vi "Device Address.vi"(10 "Device":T2=enum."V7") -> (2 "Address (all reqd.)":T1, 3 "Channel Name":string)   [LabVIEW 2011]
uses:
  Valve_Pump.ctl
  ADAM Client/Sub VIs/ADAM Controls/Address.ctl
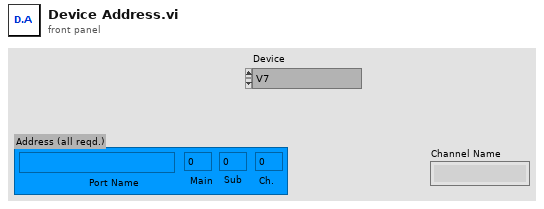
[diagram p1: front panel]
types:
  T1 = typedef "Address.ctl" = cluster{"Main":i32, "Ch.":i32, "Sub":i32, "Port Name":string}
  T2 = typedef "Valve_Pump.ctl" = enum16{"Main Rack Power", "Pump Power", "Valve Power", "V4", "V5", "V6", "V7", "V8", "V9", "V10", "V11", "V12", "V13", "V14", "V15", "V18", "V19", "V20", "V21", "V22", "V23", "V24", "V25", "V26", "V27", "V28", "V29", "V30", "V31", "V32", "V33", "V34", "Pump A", "Pump B", "Pump C", "Pump D"}
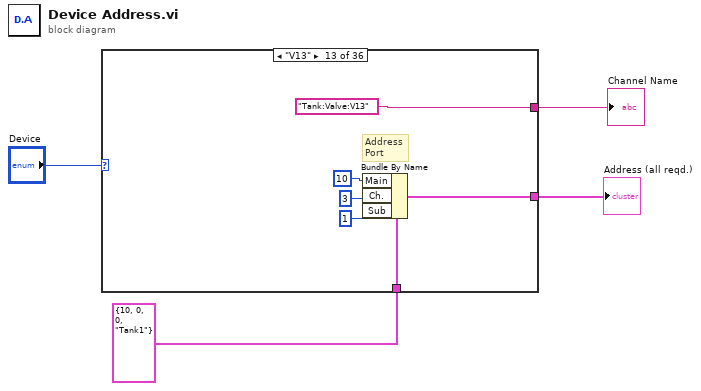
[diagram p0: block diagram]
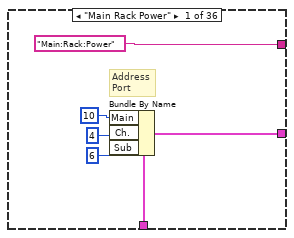
[diagram p2: hidden frame]
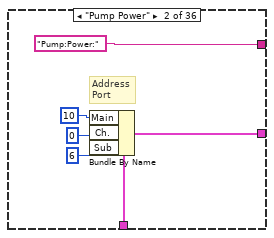
[diagram p3: hidden frame]
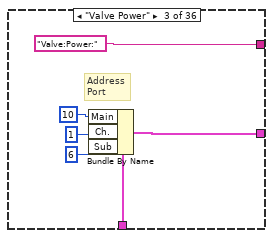
[diagram p4: hidden frame]
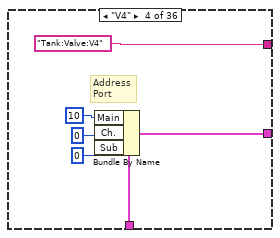
[diagram p5: hidden frame]
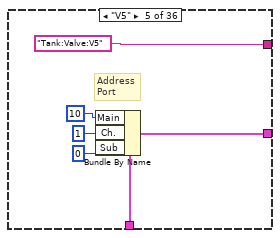
[diagram p6: hidden frame]
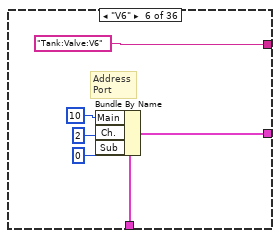
[diagram p7: hidden frame]
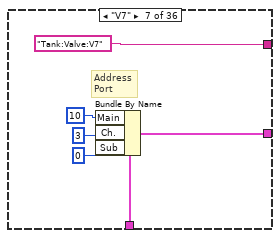
[diagram p8: hidden frame]
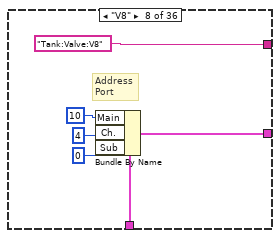
[diagram p9: hidden frame]
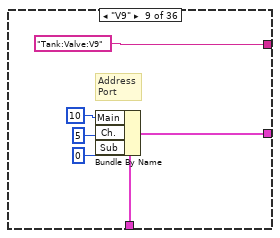
[diagram p10: hidden frame]
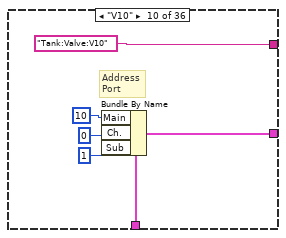
[diagram p11: hidden frame]
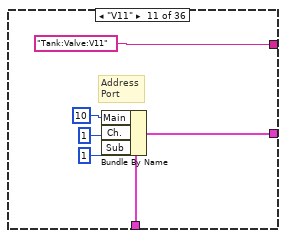
[diagram p12: hidden frame]
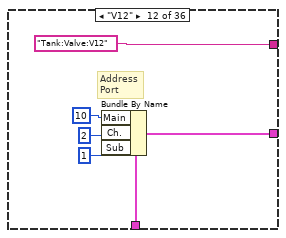
[diagram p13: hidden frame]
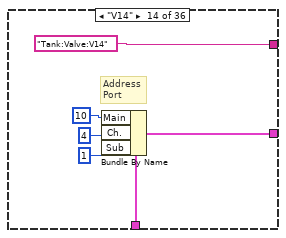
[diagram p14: hidden frame]
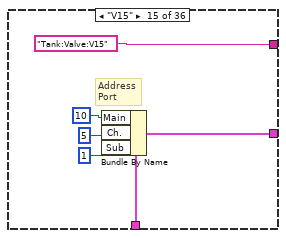
[diagram p15: hidden frame]
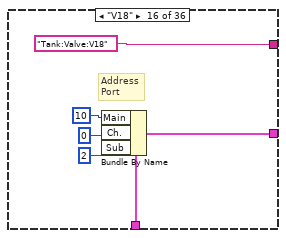
[diagram p16: hidden frame]
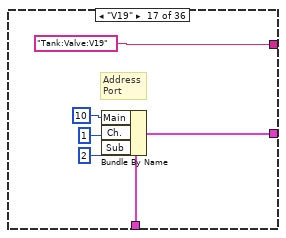
[diagram p17: hidden frame]
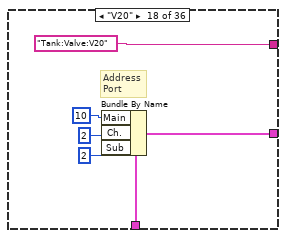
[diagram p18: hidden frame]
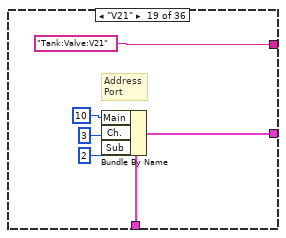
[diagram p19: hidden frame]
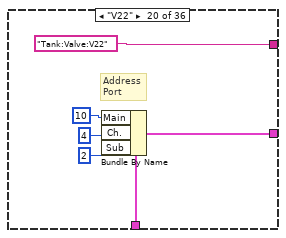
[diagram p20: hidden frame]
diagram:
  n1 = case shown="\"V13\"" "Device" {
    tunnel: T1 {"Main"=10, "Ch."=0, "Sub"=0, "Port Name"="Tank1"} ("Address (all reqd.)") -> [w10 w16 w22 w28 w34 w40 w46 w52 w58 w64 w70 w76 w82 w88 w94 w100 w106 w112 w118 w124 w130 w136 w142 w148 w154 w160 w166 w172 w178 w184 w190 w196 w202 w208 w214 w220]
    tunnel: [w6 w12 w18 w24 w30 w36 w42 w48 w54 w60 w66 w72 w78 w84 w90 w96 w102 w108 w114 w120 w126 w132 w138 w144 w150 w156 w162 w168 w174 w180 w186 w192 w198 w204 w210 w216] -> w2
    tunnel: ["Main:Rack:Power" ("Channel Name") "Pump:Power:" ("Channel Name") "Valve:Power:" ("Channel Name") "Tank:Valve:V4" ("Channel Name") "Tank:Valve:V5" ("Channel Name") "Tank:Valve:V6" ("Channel Name") "Tank:Valve:V7" ("Channel Name") "Tank:Valve:V8" ("Channel Name") "Tank:Valve:V9" ("Channel Name") "Tank:Valve:V10" ("Channel Name") "Tank:Valve:V11" ("Channel Name") "Tank:Valve:V12" ("Channel Name") "Tank:Valve:V13" ("Channel Name") "Tank:Valve:V14" ("Channel Name") "Tank:Valve:V15" ("Channel Name") "Tank:Valve:V18" ("Channel Name") "Tank:Valve:V19" ("Channel Name") "Tank:Valve:V20" ("Channel Name") "Tank:Valve:V21" ("Channel Name") "Tank:Valve:V22" ("Channel Name") "Tank:Valve:V23" ("Channel Name") "Tank:Valve:V24" ("Channel Name") "Tank:Valve:V25" ("Channel Name") "Tank:Valve:V26" ("Channel Name") "Tank:Valve:V27" ("Channel Name") "Tank:Valve:V28" ("Channel Name") "Tank:Valve:V29" ("Channel Name") "Tank:Valve:V30" ("Channel Name") "Tank:Valve:V31" ("Channel Name") "Tank:Valve:V32" ("Channel Name") "Tank:Valve:V33" ("Channel Name") "Tank:Valve:V34" ("Channel Name") "Tank:Valve:Pump A" ("Channel Name") "Tank:Valve:Pump B" ("Channel Name") "Tank:Valve:Pump C" ("Channel Name") "Tank:Valve:Pump D" ("Channel Name")] -> w1
    frame "Main Rack Power" {
      # "Address \nPort"
      n2 = Bundle By Name(cluster=w10, "Main"=10, "Ch."=4, "Sub"=6) -> (w6:T1)
    }
    frame "Pump Power" {
      # "Address \nPort"
      n3 = Bundle By Name(cluster=w16, "Main"=10, "Ch."=0, "Sub"=6) -> (w12:T1)
    }
    frame "Valve Power" {
      # "Address \nPort"
      n4 = Bundle By Name(cluster=w22, "Main"=10, "Ch."=1, "Sub"=6) -> (w18:T1)
    }
    frame "V4" {
      # "Address \nPort"
      n5 = Bundle By Name(cluster=w28, "Main"=10, "Ch."=0, "Sub"=0) -> (w24:T1)
    }
    frame "V5" {
      # "Address \nPort"
      n6 = Bundle By Name(cluster=w34, "Main"=10, "Ch."=1, "Sub"=0) -> (w30:T1)
    }
    frame "V6" {
      # "Address \nPort"
      n7 = Bundle By Name(cluster=w40, "Main"=10, "Ch."=2, "Sub"=0) -> (w36:T1)
    }
    frame "V7" {
      # "Address \nPort"
      n8 = Bundle By Name(cluster=w46, "Main"=10, "Ch."=3, "Sub"=0) -> (w42:T1)
    }
    frame "V8" {
      # "Address \nPort"
      n9 = Bundle By Name(cluster=w52, "Main"=10, "Ch."=4, "Sub"=0) -> (w48:T1)
    }
    frame "V9" {
      # "Address \nPort"
      n10 = Bundle By Name(cluster=w58, "Main"=10, "Ch."=5, "Sub"=0) -> (w54:T1)
    }
    frame "V10" {
      # "Address \nPort"
      n11 = Bundle By Name(cluster=w64, "Main"=10, "Ch."=0, "Sub"=1) -> (w60:T1)
    }
    frame "V11" {
      # "Address \nPort"
      n12 = Bundle By Name(cluster=w70, "Main"=10, "Ch."=1, "Sub"=1) -> (w66:T1)
    }
    frame "V12" {
      # "Address \nPort"
      n13 = Bundle By Name(cluster=w76, "Main"=10, "Ch."=2, "Sub"=1) -> (w72:T1)
    }
    frame "V13" {
      # "Address \nPort"
      n14 = Bundle By Name(cluster=w82, "Main"=10, "Ch."=3, "Sub"=1) -> (w78:T1)
    }
    frame "V14" {
      # "Address \nPort"
      n15 = Bundle By Name(cluster=w88, "Main"=10, "Ch."=4, "Sub"=1) -> (w84:T1)
    }
    frame "V15" {
      # "Address \nPort"
      n16 = Bundle By Name(cluster=w94, "Main"=10, "Ch."=5, "Sub"=1) -> (w90:T1)
    }
    frame "V18" {
      # "Address \nPort"
      n17 = Bundle By Name(cluster=w100, "Main"=10, "Ch."=0, "Sub"=2) -> (w96:T1)
    }
    frame "V19" {
      # "Address \nPort"
      n18 = Bundle By Name(cluster=w106, "Main"=10, "Ch."=1, "Sub"=2) -> (w102:T1)
    }
    frame "V20" {
      # "Address \nPort"
      n19 = Bundle By Name(cluster=w112, "Main"=10, "Ch."=2, "Sub"=2) -> (w108:T1)
    }
    frame "V21" {
      # "Address \nPort"
      n20 = Bundle By Name(cluster=w118, "Main"=10, "Ch."=3, "Sub"=2) -> (w114:T1)
    }
    frame "V22" {
      # "Address \nPort"
      n21 = Bundle By Name(cluster=w124, "Main"=10, "Ch."=4, "Sub"=2) -> (w120:T1)
    }
    frame "V23" {
      # "Address \nPort"
      n22 = Bundle By Name(cluster=w130, "Main"=10, "Ch."=5, "Sub"=2) -> (w126:T1)
    }
    frame "V24" {
      # "Address \nPort"
      n23 = Bundle By Name(cluster=w136, "Main"=10, "Ch."=0, "Sub"=3) -> (w132:T1)
    }
    frame "V25" {
      # "Address \nPort"
      n24 = Bundle By Name(cluster=w142, "Main"=10, "Ch."=1, "Sub"=3) -> (w138:T1)
    }
    frame "V26" {
      # "Address \nPort"
      n25 = Bundle By Name(cluster=w148, "Main"=10, "Ch."=2, "Sub"=3) -> (w144:T1)
    }
    frame "V27" {
      # "Address \nPort"
      n26 = Bundle By Name(cluster=w154, "Main"=10, "Ch."=3, "Sub"=3) -> (w150:T1)
    }
    frame "V28" {
      # "Address \nPort"
      n27 = Bundle By Name(cluster=w160, "Main"=10, "Ch."=4, "Sub"=3) -> (w156:T1)
    }
    frame "V29" {
      # "Address \nPort"
      n28 = Bundle By Name(cluster=w166, "Main"=10, "Ch."=5, "Sub"=3) -> (w162:T1)
    }
    frame "V30" {
      # "Address \nPort"
      n29 = Bundle By Name(cluster=w172, "Main"=10, "Ch."=0, "Sub"=4) -> (w168:T1)
    }
    frame "V31" {
      # "Address \nPort"
      n30 = Bundle By Name(cluster=w178, "Main"=10, "Ch."=1, "Sub"=4) -> (w174:T1)
    }
    frame "V32" {
      # "Address \nPort"
      n31 = Bundle By Name(cluster=w184, "Main"=10, "Ch."=2, "Sub"=4) -> (w180:T1)
    }
    frame "V33" {
      # "Address \nPort"
      n32 = Bundle By Name(cluster=w190, "Main"=10, "Ch."=3, "Sub"=4) -> (w186:T1)
    }
    frame "V34" {
      # "Address \nPort"
      n33 = Bundle By Name(cluster=w196, "Main"=10, "Ch."=4, "Sub"=4) -> (w192:T1)
    }
    frame "Pump A" {
      # "Address \nPort"
      n34 = Bundle By Name(cluster=w202, "Main"=10, "Ch."=0, "Sub"=5) -> (w198:T1)
    }
    frame "Pump B" {
      # "Address \nPort"
      n35 = Bundle By Name(cluster=w208, "Main"=10, "Ch."=1, "Sub"=5) -> (w204:T1)
    }
    frame "Pump C" {
      # "Address \nPort"
      n36 = Bundle By Name(cluster=w214, "Main"=10, "Ch."=2, "Sub"=5) -> (w210:T1)
    }
    frame "Pump D" {
      # "Address \nPort"
      n37 = Bundle By Name(cluster=w220, "Main"=10, "Ch."=3, "Sub"=5) -> (w216:T1)
    }
  }
  "Address (all reqd.)" <- w2
  "Channel Name" <- w1
